vi "G#Object_NewDebugObject.vi"(0 "reference in":refnum<class "G#Object.lvclass">, 5 "error in (no error)":errorcluster) -> (14 "reference out":refnum<class "G#Object.lvclass">, 19 "error out":errorcluster)   [LabVIEW 2020, in "G#Object.lvclass"]
doc: "Creates the object as a debug object."
uses:
  G#Object.lvclass
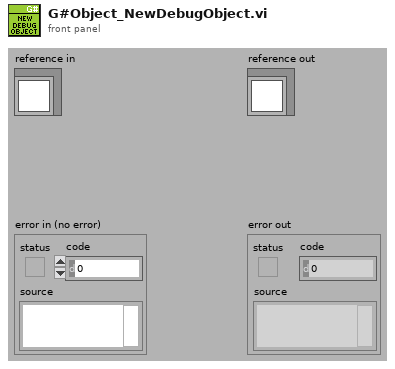
[diagram p1: front panel]
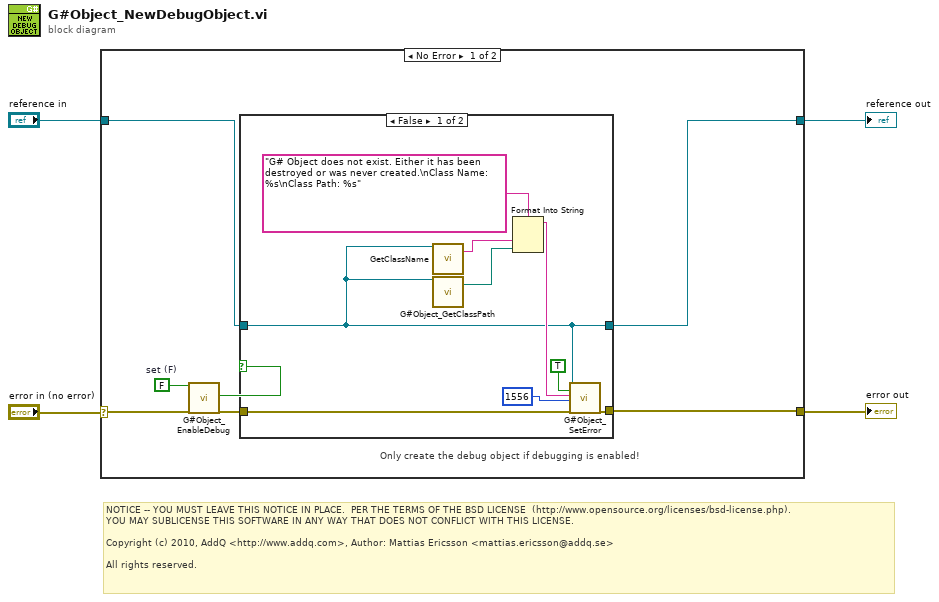
[diagram p0: block diagram]
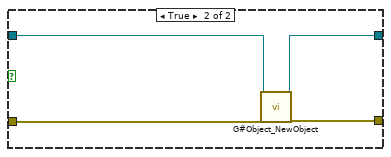
[diagram p2: hidden frame]
diagram:
  # "NOTICE -- YOU MUST LEAVE THIS NOTICE IN PLACE.  PER THE TERMS OF THE BSD LICENSE  (http://www.opensource.org/licenses/bsd-license.php).\nYOU MAY SUBLICENSE THIS SOFTWARE IN ANY WAY THAT DOES NOT CONFLICT WITH THIS LICENSE.\n\nCopyright (c) 2010, AddQ <http://www.addq.com>, Author: Mattias Ericsson <mattias.ericsson@addq.se>\n\nAll rights reserved."
  n1 = case shown="No Error" "error in (no error)" {
    selector: "error in (no error)" -> [w11 w26]
    tunnel: [w5 w26] -> w3
    tunnel: [w7 w25] -> w1
    tunnel: "reference in" -> [w8 w25]
    frame No Error {
      w10 = FALSE  # set (F)
      # "Only create the debug object if debugging is enabled!"
      n2 = call "G#Object_EnableDebug.vi"("set (F)"=w10, "error in (no error)"=w11) -> ("enabled"=w6:bool, "error out"=w9:errorcluster)  [unwired: 15 in, 1 out]
      n3 = case shown="False" w6 {
        tunnel: w9 -> [w19 w24]
        tunnel: w8 -> [w13 w22]
        tunnel: [w13 w21] -> w7
        tunnel: [w20 w23] -> w5
        frame False {
          n4 = call-dynamic "GetClassName.vi"("reference in"=w13) -> ("class name"=w12:string)  [unwired: 14 in, 4 out]
          n5 = call-dynamic "G#Object_GetClassPath.vi"("reference in"=w13) -> ("class path"=w14:path)  [unwired: 16 in, 2 out]
          n6 = Format Into String(format string="G# Object does not exist. Either it has been destroyed or was never created.\nClass Name: %s\nClass Path: %s", w12, w14) -> (resulting string=w16:string)  [unwired: 2 in, 1 out]
          n7 = call "G#Object_SetError.vi"("reference in"=w13, "error (F)"=TRUE, "source"=w16, "code"=1556, "error in (no error)"=w19) -> ("error out"=w20:errorcluster)  [unwired: 14 in]
        }
        frame True {
          n8 = call "G#Object_NewObject.vi"("reference in"=w22, "error in (no error)"=w24) -> ("reference out"=w21:refnum<class "G#Object.lvclass">, "error out"=w23:errorcluster)  [unwired: 15 in, 1 out]
        }
      }
    }
    frame Error {
    }
  }
  "error out" <- w3
  "reference out" <- w1
